vi "SLSC Command Enum Constant.vi"(0 "Enum Value":i32=-1, 5 "Option on Reset?":bool) -> (4 "Array":T1[](array[typedef]), 6 "String Enums":cluster{"name":string, "string enums":string}[](array[cluster]), 8 "string enum":string, 10 "String":string, 14 "string enums":string)   [LabVIEW 2017, in "SLSC Tree Control.lvlib"]
uses:
  SLSC Tree Control.lvlib
  SLSC EDS API/JSON parsing/enum.ctl
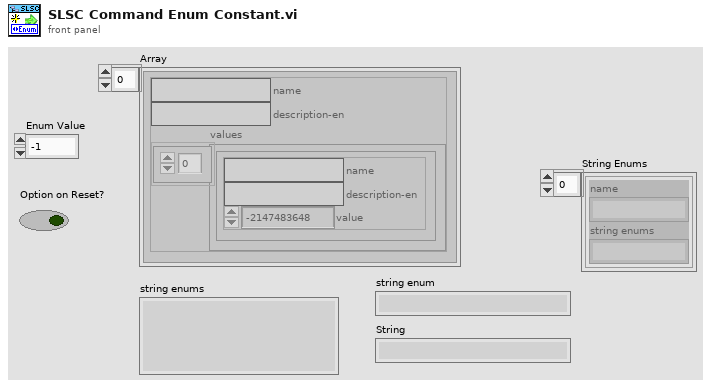
[diagram p1: front panel]
types:
  T1 = typedef "enum.ctl" = cluster{"name":string, "description-en":string, "values":cluster{"name":string, "description-en":string, "value":i32}[]}
  T2 = cluster{"name":string, "description-en":string, "value":i32}[]
  T3 = cluster{"Name":string, "Enum Names":string[], "Enum Values":i32[]}[]
  T4 = cluster{"name":string, "description-en":string, "value":i32}
  T5 = cluster{"Name":string, "Enum Names":string[], "Enum Values":i32[]}
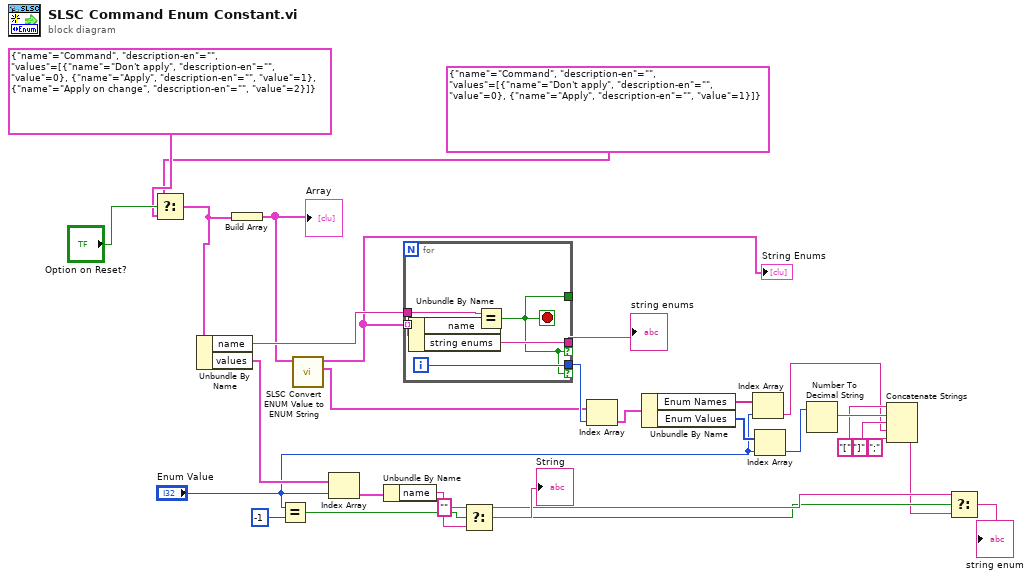
[diagram p0: block diagram]
diagram:
  w23 = "" ("t")
  n1 = Select(t=T1 {"name"="Command", "description-en"="", "values"=[{"name"="Don't apply", "description-en"="", "value"=0}, {"name"="Apply", "description-en"="", "value"=1}]} ("enum"), s="Option on Reset?", f=T1 {"name"="Command", "description-en"="", "values"=[{"name"="Don't apply", "description-en"="", "value"=0}, {"name"="Apply", "description-en"="", "value"=1}, {"name"="Apply on change", "description-en"="", "value"=2}]} ("enum")) -> (s? t:f=w2:T1)
  n2 = Unbundle By Name(w2) -> ("name"=w28:string, "values"=w27:T2)
  n3 = Build Array(w2) -> (w18:T1[])
  "Array" <- w18
  n4 = Equal?(x="Enum Value", y=-1) -> (x = y?=w22:bool)
  n5 = call "SLSC Convert ENUM Value to ENUM String.vi"("Enums"=w18) -> ("Cluster Enums"=w17:T3, "String Enums"=w5:cluster{"name":string, "string enums":string}[])  [unwired: 9 in]
  "String Enums" <- w5
  n6 = Index Array(array=w27, index="Enum Value") -> (element=w20:T4)
  n7 = Unbundle By Name(w20) -> ("name"=w25:string)
  n8 = for {
    tunnel: w5 -> [w35] mode=indexing
    tunnel: w28 -> [w33]
    tunnel: [w32] -> w29 if=w30
    tunnel: [w30] -> _
    tunnel: [w31] -> w19 if=w30
    i -> [w31]
    stop <- w30 stop-if-true
    n9 = Unbundle By Name(w35) -> ("name"=w34:string, "string enums"=w32:string)
    n10 = Equal?(x=w33, y=w34) -> (x = y?=w30:bool)
  }
  "string enums" <- w29
  n11 = Select(t=w23, s=w22, f=w25) -> (s? t:f=→"String":string)
  n12 = Index Array(array=w17, index=w19) -> (element=w16:T5)
  n13 = Unbundle By Name(w16) -> ("Enum Names"=w11:string[], "Enum Values"=w10:i32[])
  n14 = Index Array(array=w11, index="Enum Value") -> (element=w8:string)
  n15 = Index Array(array=w10, index="Enum Value") -> (element=w7:i32)
  n16 = Number To Decimal String(number=w7) -> (decimal integer string=w15:string)  [unwired: 1 in]
  n17 = Concatenate Strings("[" ("string"), w15, "]" ("string"), w8, ";" ("string")) -> (w6:string)
  n18 = Select(t=w23, s=w22, f=w6) -> (s? t:f=→"string enum":string)
